vi "FGA Write To Log File.vi"(0 "LogData":T1) -> ()   [LabVIEW 2009]
uses:
  LogData.ctl
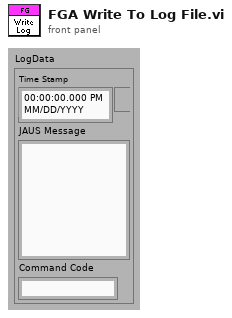
[diagram p1: front panel]
types:
  T1 = typedef "LogData.ctl" = cluster{"Time Stamp":timestamp, "JAUS Message":string, "Command Code":string}
  T2 = enum16{"open", "replace", "create", "open or create", "replace or create", "replace or create with confirmation"}
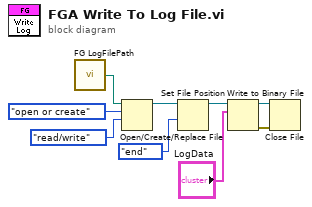
[diagram p0: block diagram]
diagram:
  n1 = call "FG LogFilePath.vi"() -> ("path out"=w9:path)  [unwired: 2 in]
  n2 = Open/Create/Replace File(file path (use dialog)=w9, operation (0:open)=T2."open or create", access (0:read/write)=enum16{"read/write", "read-only", "write-only"}."read/write") -> (refnum out=w6:refnum<file>)  [unwired: 3 in, 2 out]
  n3 = Set File Position(refnum=w6, from (0:start)=enum16{"start", "end", "current"}."end") -> (refnum out=w2:refnum<file>)  [unwired: 2 in, 1 out]
  n4 = Write to Binary File(file (use dialog)=w2, data="LogData") -> (refnum out=w3:refnum<file>, error out=w4:errorcluster)  [unwired: 4 in, 1 out]
  n5 = Close File(refnum=w3, error in=w4) -> ()  [unwired: 2 out]
